vi "Desired Value Page.vi"(8 "error in (no error)":errorcluster, 11 "Node Ptr":T3 format="%.0x") -> (0 "error out":errorcluster)   [LabVIEW 2021, in "NI 272x Resistive Simulation Custom Device Configuration.lvlib"]
uses:
  NI 272x Resistive Simulation Custom Device Configuration.lvlib
  Program Files/National Instruments/LabVIEW 2021/vi.lib/NI VeriStand/Custom Device API/Custom Device Item Ref.ctl
  Program Files/National Instruments/LabVIEW 2021/instr.lib/ni272xReferenceVIs/ni272xReferenceVIs.llb/ni272x Callendar-Van Dusen RTD Parameters.ctl
  Controls/Channel Mode.ctl
  Globals/Names.vi
  Program Files/National Instruments/LabVIEW 2021/vi.lib/NI VeriStand/Custom Device API/Get Item Property (U16).vi
  Program Files/National Instruments/LabVIEW 2021/vi.lib/NI VeriStand/Custom Device API/Get Item Property (I32).vi
  Program Files/National Instruments/LabVIEW 2021/vi.lib/NI VeriStand/Custom Device API/Set Item Property (I32).vi
  Program Files/National Instruments/LabVIEW 2021/vi.lib/NI VeriStand/Custom Device API/Set Item Property (U16).vi
  Program Files/National Instruments/LabVIEW 2021/vi.lib/NI VeriStand/Custom Device API/Custom Device API.lvlib
  NI 272x Resistive Simulation Custom Device Shared.lvlib
panel:
  out "Units":string
  in  "Default Value":dbl
  in  "Mode":T1
  in  "Channel #":i32 min=0
  in  "Callendar-Van Dusen RTD parameters":T2={"A"=0.00139999995008111, "B"=0.00023700000019744039, "C"=9.899999753315569e-08, "R0"=1000.0}
  in  "Header":cluster{"Section Name":string}={"Section Name"="Desired Hardware Channel Value"}
  in  "Description":string
  in  "Name":string
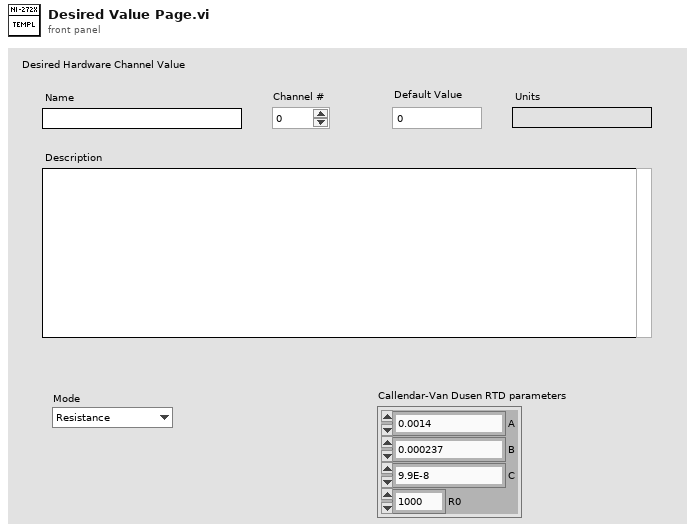
[diagram p1: front panel]
types:
  T1 = typedef "NI 272x Resistive Simulation Custom Device Shared.lvlib/Channel Mode.ctl" = enum16{"Resistance", "RTD Temperature"}
  T2 = typedef "ni272x Callendar-Van Dusen RTD Parameters.ctl" = cluster{"A":dbl, "B":dbl, "C":dbl, "R0":dbl}
  T3 = typedef "Custom Device API.lvlib/Custom Device Item Ref.ctl" = u64
  T4 = typedef "Custom Device API.lvlib/Custom Device Channel.ctl" = cluster{"Type":T5, "Units":string, "Default Value":dbl, "Faultable":bool, "Scalable":bool}
  T5 = typedef "Custom Device API.lvlib/Custom Device Channel Type.ctl" = enum16{"Input", "Output"}
  T6 = typedef "Custom Device API.lvlib/Custom Device Item Info.ctl" = cluster{"Name":string, "Is Channel":bool, "GUID":string, "Is Waveform":bool}
  T7 = typedef "Custom Device API.lvlib/Custom Device Commands.ctl" = enum16{"Default", "Item renamed", "Shutdown", "Dynamic button pressed"}
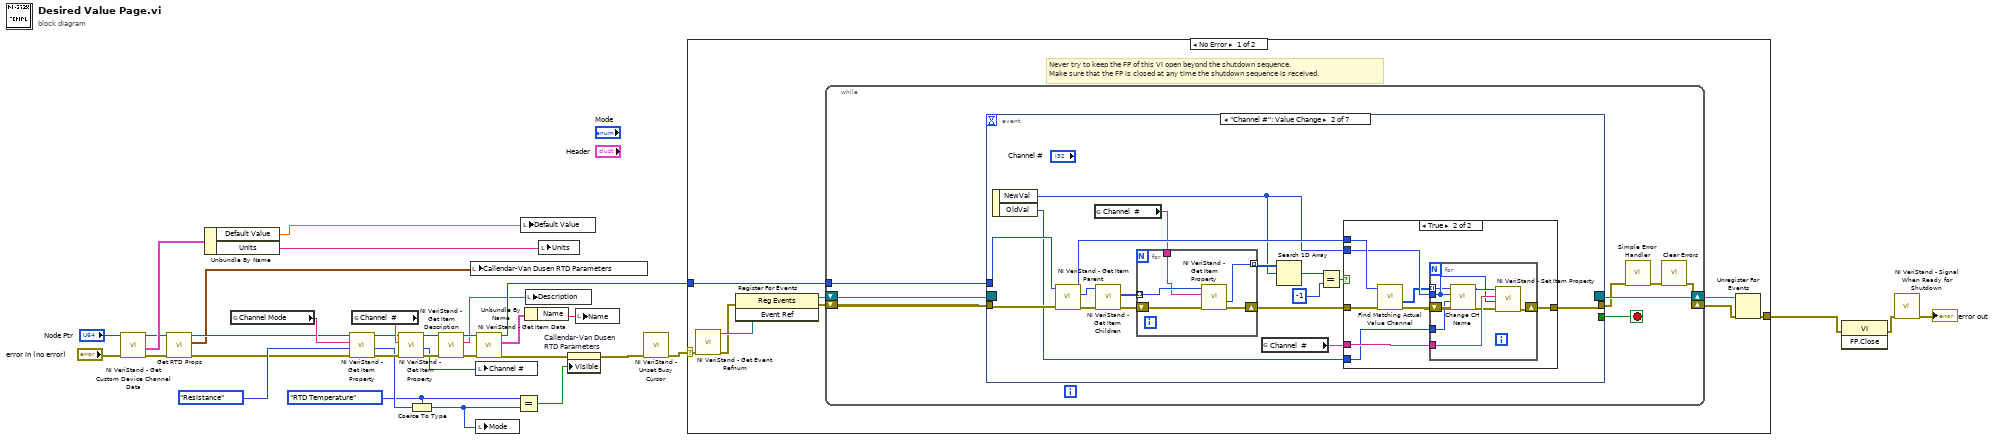
[diagram p0: block diagram]
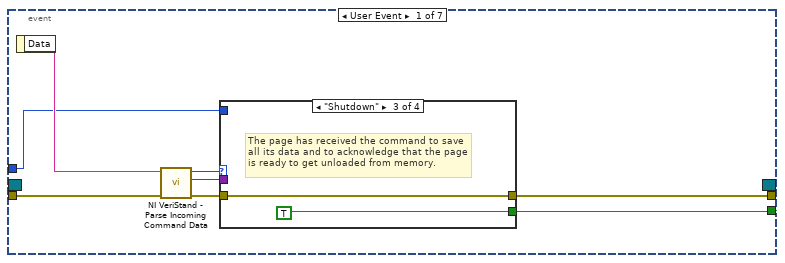
[diagram p2: hidden frame]
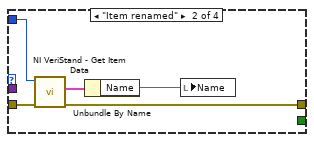
[diagram p4: hidden frame]
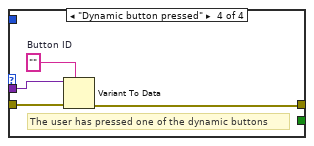
[diagram p5: hidden frame]
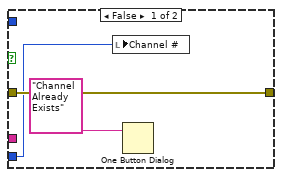
[diagram p6: hidden frame]
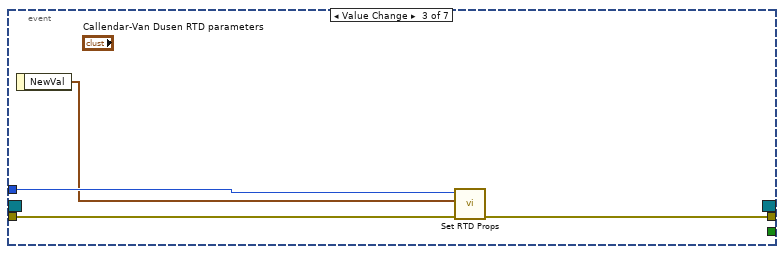
[diagram p7: hidden frame]
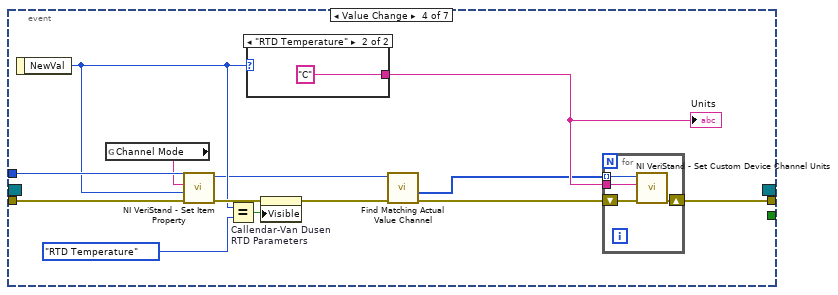
[diagram p8: hidden frame]
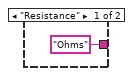
[diagram p9: hidden frame]
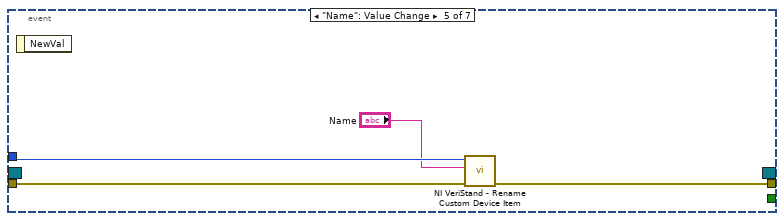
[diagram p10: hidden frame]
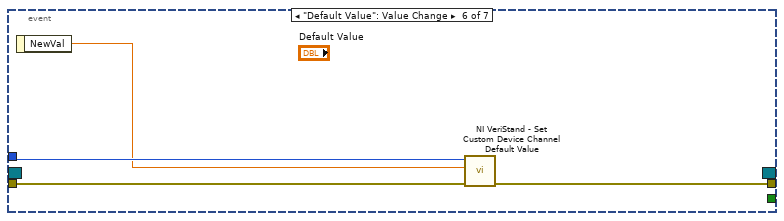
[diagram p11: hidden frame]
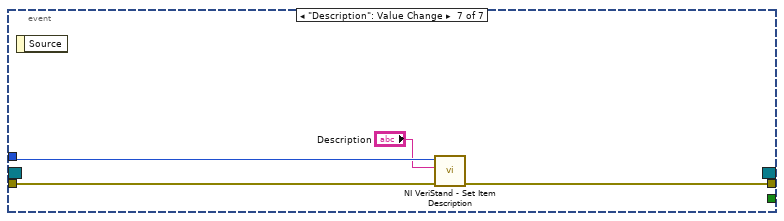
[diagram p12: hidden frame]
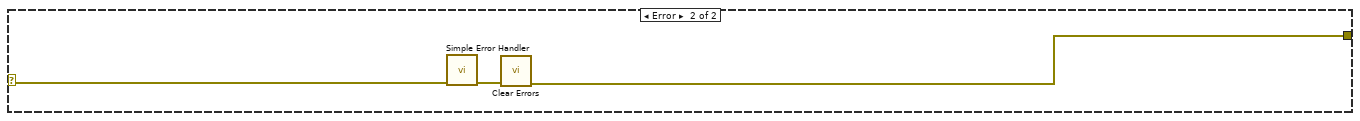
[diagram p13: hidden frame]
diagram:
  w13 = Channel_Mode."RTD Temperature" ("Mode")
  n1 = call "NI VeriStand - Get Custom Device Channel Data.vi"("error in (no error)"="error in (no error)", "Channel Ref in"="Node Ptr") -> ("error out"=w10:errorcluster, "Channel"=w8:T4, "Channel Ref out"=w3:T3)  [unwired: 4 in, 3 out]
  n2 = call "Get RTD Props.vi"("error in (no error)"=w10, "Item Ref in"=w3) -> ("error out"=w4:errorcluster, "temp param"=w1:T2, "Item Ref out"=w2:T3)  [unwired: 7 in]
  n3 = Unbundle By Name(w8) -> ("Default Value"=w5:dbl, "Units"=w7:string)
  n4 = global read "Names.vi" "Channel Mode"() -> (w16:string)
  n5 = call-poly "NI VeriStand - Get Item Property.vi"("error in (no error)"=w4, "Default Value"=Channel_Mode."Resistance" ("Mode"), "Property Name"=w16, "Item Ref in"=w2) -> ("error out"=w17:errorcluster, "Value"=w15:u16, "Item Ref out"=w18:T3)  [unwired: 4 in, 1 out]
  n6 = global read "Names.vi" "Channel  #"() -> (w20:string)
  n7 = call-poly "NI VeriStand - Get Item Property.vi"("error in (no error)"=w17, "Property Name"=w20, "Item Ref in"=w18) -> ("error out"=w21:errorcluster, "Value"=w19:i32, "Item Ref out"=w22:T3)  [unwired: 5 in, 1 out]
  n8 = Coerce To Type(0:w15, 1:w13) -> (2:w12:T1)
  n9 = call "NI VeriStand - Get Item Description.vi"("error in (no error)"=w21, "Item Ref in"=w22) -> ("error out"=w25:errorcluster, "Description"=w26:string, "Item Ref out"=w27:T3)  [unwired: 7 out]
  n10 = local write "Callendar-Van Dusen RTD parameters"(w1) -> ()
  n11 = local write "Channel #"(w19) -> ()
  n12 = local write "Mode"(w12) -> ()
  n13 = call "NI VeriStand - Get Item Data.vi"("error in (no error)"=w25, "Item Ref in"=w27) -> ("error out"=w14:errorcluster, "Item Info"=w24:T6, "Item Ref out"=w29:T3)  [unwired: 7 out]
  n14 = Equal?(x=w13, y=w12) -> (x = y?=w11:bool)
  n15 = local write "Default Value"(w5) -> ()
  n16 = Unbundle By Name(w24) -> ("Name"=w23:string)
  n17 = local write "Description"(w26) -> ()
  n18 = local write "Units"(w7) -> ()
  n19 = property on="Callendar-Van Dusen RTD Parameters" class="Clust (strict)"(error in=w14, "Visible"=w11) -> (error out=w31:errorcluster)  [unwired: 1 in, 1 out]
  n20 = local write "Name"(w23) -> ()
  n21 = call "NI VeriStand - Unset Busy Cursor.vi"("error in (no error)"=w31) -> ("error out"=w30:errorcluster)  [unwired: 10 out]
  n22 = case shown="No Error" w30 {
    selector: w30 -> [w36 w149]
    tunnel: [w41 w147] -> w34
    tunnel: w29 -> [w37 _]
    frame No Error {
      # "Never try to keep the FP of this VI open beyond the shutdown sequence.\nMake sure that the FP is closed at any time the shutdown sequence is received."
      n23 = call "NI VeriStand - Get Event Refnum.vi"("error in (no error)"=w36) -> ("error out"=w35:errorcluster, "Event Ref"=w40:refnum<user-event>)  [unwired: 9 out]
      n24 = register-events(error in=w35, w40) -> (reference out=w38:refnum<event-registration>, error out=w39:errorcluster)  [unwired: 1 in]
      n25 = while {
        tunnel: w37 -> [w47]
        shift-right: [w45] -> w42
        shift-left: w39 -> [w50]
        shift-right: [w51] -> w43
        shift-left: w38 -> [w49]
        stop <- w48 stop-if-true
        n26 = event shown="[1] \"Channel #\": Value Change" {
          selector: w49 -> [_ _ _ _ _ _ _]
          dyn-events: [_ _ _ _ _ _ _] -> w51
          timeout: _ -> [_ _ _ _ _ _ _]
          tunnel: w50 -> [w59 w78 w116 w128 w138 w142 w145]
          tunnel: [w55 _ _ _ _ _ _] -> w48
          tunnel: [w54 w74 w115 w122 w135 w140 w144] -> w44
          tunnel: w47 -> [w53 w77 w114 w127 w137 w141 w146]
          event User Event {
            n27 = event-data() -> ("Data"=w58:string)  [unwired: 1 out]
            n28 = call "NI VeriStand - Parse Incoming Command Data.vi"("error in (no error)"=w59, "Incoming data"=w58) -> ("error out"=w57:errorcluster, "Outgoing data"=w52:variant, "Action"=w56:T7)  [unwired: 7 out]
            n29 = case shown="\"Shutdown\"" w56 {
              tunnel: w57 -> [w60 w65 w66 w71]
              tunnel: [_ _ TRUE _] -> w55
              tunnel: [w60 w62 w66 w68] -> w54
              tunnel: w53 -> [_ w64 _ _]
              tunnel: w52 -> [_ _ _ w70]
              frame "Default", Default {
              }
              frame "Item renamed" {
                n30 = call "NI VeriStand - Get Item Data.vi"("error in (no error)"=w65, "Item Ref in"=w64) -> ("error out"=w62:errorcluster, "Item Info"=w63:T6)  [unwired: 8 out]
                n31 = Unbundle By Name(w63) -> ("Name"=w61:string)
                n32 = local write "Name"(w61) -> ()
              }
              frame "Shutdown" {
                # "The page has received the command to save all its data and to acknowledge that the page is ready to get unloaded from memory."
              }
              frame "Dynamic button pressed" {
                w69 = ""  # Button ID
                # "The user has pressed one of the dynamic buttons"
                n33 = Variant To Data(error in=w71, type=w69, Variant=w70) -> (error out=w68:errorcluster)  [unwired: 1 out]
              }
            }
          }
          event "Channel #": Value Change {
            n34 = event-data() -> ("NewVal"=w76:i32, "OldVal"=w75:i32)  [unwired: 1 out]
            n35 = call "NI VeriStand - Get Item Parent.vi"("error in (no error)"=w78, "Item Ref in"=w77) -> ("error out"=w79:errorcluster, "Parent Ref"=w80:T3, "Item Ref out"=w88:T3)  [unwired: 6 in, 1 out]
            n36 = global read "Names.vi" "Channel  #"() -> (w72:string)
            n37 = call "NI VeriStand - Get Item Children.vi"("error in (no error)"=w79, "Item Ref in"=w80) -> ("error out"=w82:errorcluster, "Child Refs"=w81:T3[])  [unwired: 6 in, 2 out]
            n38 = for {
              tunnel: w81 -> [w110] mode=indexing
              shift-right: [w111] -> w87
              shift-left: w82 -> [w112]
              tunnel: [w109] -> w83 mode=indexing
              tunnel: w72 -> [w108]
              n39 = call-poly "NI VeriStand - Get Item Property.vi"("error in (no error)"=w112, "Property Name"=w108, "Item Ref in"=w110) -> ("error out"=w111:errorcluster, "Value"=w109:i32)  [unwired: 5 in, 2 out]
            }
            n40 = global read "Names.vi" "Channel  #"() -> (w73:string)
            n41 = Search 1D Array(1D array=w83, element=w76) -> (index of element=w84:i32)  [unwired: 1 in]
            n42 = Equal?(x=w84, y=-1) -> (x = y?=w86:bool)
            n43 = case shown="True" w86 {
              tunnel: w87 -> [w91 w97]
              tunnel: w88 -> [_ w96]
              tunnel: w73 -> [_ w98]
              tunnel: w76 -> [_ w95]
              tunnel: [w91 w99] -> w74
              tunnel: w75 -> [w89 w92]
              frame False {
                n44 = local write "Channel #"(w89) -> ()
                n45 = One Button Dialog(message="Channel Already Exists") -> ()  [unwired: 1 in, 1 out]
              }
              frame True {
                n46 = call "Find Matching Actual Value Channel.vi"("error in (no error)"=w97, "Desired item ref in"=w96) -> ("error out"=w94:errorcluster, "Refs (desired first)"=w93:T3[])  [unwired: 4 in, 4 out]
                n47 = for {
                  tunnel: w98 -> [w106]
                  shift-right: [w107] -> w99
                  shift-left: w94 -> [w104]
                  tunnel: w95 -> [w102]
                  tunnel: w93 -> [w101] mode=indexing
                  tunnel: w92 -> [w100]
                  n48 = call "Change CH Name.vi"("error in (no error)"=w104, "Old #"=w100, "New #"=w102, "Node Ptr"=w101) -> ("error out"=w105:errorcluster, "Node Ptr out"=w103:T3)  [unwired: 6 in]
                  n49 = call-poly "NI VeriStand - Set Item Property.vi"("error in (no error)"=w105, "Value"=w102, "Property Name"=w106, "Item Ref in"=w103) -> ("error out"=w107:errorcluster)  [unwired: 5 in, 2 out]
                }
              }
            }
          }
          event Value Change {
            n50 = event-data() -> ("NewVal"=w113:T2)  [unwired: 1 out]
            n51 = call "Set RTD Props.vi"("error in (no error)"=w116, "temp param"=w113, "Item Ref in"=w114) -> ("error out"=w115:errorcluster)  [unwired: 7 in, 1 out]
          }
          event Value Change {
            n52 = event-data() -> ("NewVal"=w121:T1)  [unwired: 1 out]
            n53 = global read "Names.vi" "Channel Mode"() -> (w126:string)
            n54 = call-poly "NI VeriStand - Set Item Property.vi"("error in (no error)"=w128, "Value"=w121, "Property Name"=w126, "Item Ref in"=w127) -> ("error out"=w125:errorcluster, "Item Ref out"=w118:T3)  [unwired: 5 in, 1 out]
            n55 = Equal?(x=w121, y=Channel_Mode."RTD Temperature" ("NewVal")) -> (x = y?=w124:bool)
            n56 = case shown="\"RTD Temperature\"" w121 {
              tunnel: ["Ohms" ("Units") "C" ("Units")] -> w120
              frame "Resistance" {
              }
              frame "RTD Temperature" {
              }
            }
            "Units" <- w120
            n57 = property on="Callendar-Van Dusen RTD Parameters" class="Clust (strict)"(error in=w125, "Visible"=w124) -> (error out=w119:errorcluster)  [unwired: 1 in, 1 out]
            n58 = call "Find Matching Actual Value Channel.vi"("error in (no error)"=w119, "Desired item ref in"=w118) -> ("Refs (desired first)"=w117:T3[])  [unwired: 4 in, 5 out]
            n59 = for {
              tunnel: w120 -> [w131]
              shift-right: [w132] -> w122
              shift-left: w119 -> [w130]
              tunnel: w117 -> [w129] mode=indexing
              n60 = call "NI VeriStand - Set Custom Device Channel Units.vi"("error in (no error)"=w130, "Units"=w131, "Channel Ref in"=w129) -> ("error out"=w132:errorcluster)  [unwired: 7 in, 1 out]
            }
          }
          event "Name": Value Change {
            n61 = event-data() -> ()  [unwired: 2 out]
            n62 = call "NI VeriStand - Rename Custom Device Item.vi"("error in (no error)"=w138, "New Name"="Name", "Item Ref in"=w137) -> ("error out"=w135:errorcluster)  [unwired: 1 in, 7 out]
          }
          event "Default Value": Value Change {
            n63 = event-data() -> ("NewVal"=w139:dbl)  [unwired: 1 out]
            n64 = call "NI VeriStand - Set Custom Device Channel Default Value.vi"("error in (no error)"=w142, "Default Value"=w139, "Channel Ref in"=w141) -> ("error out"=w140:errorcluster)  [unwired: 7 in, 1 out]
          }
          event "Description": Value Change {
            n65 = event-data() -> ()  [unwired: 2 out]
            n66 = call "NI VeriStand - Set Item Description.vi"("error in (no error)"=w145, "Description"="Description", "Item Ref in"=w146) -> ("error out"=w144:errorcluster)  [unwired: 8 out]
          }
        }
        n67 = call <vilib>:"Simple Error Handler.vi"("error in (no error)"=w44) -> ("error out"=w46:errorcluster)  [unwired: 1 in, 7 out]
        n68 = call <vilib>:"Clear Errors.vi"("error in (no error)"=w46) -> ("error out"=w45:errorcluster)  [unwired: 1 in, 5 out]
      }
      n69 = Unregister For Events(event registration refnum=w43, error in=w42) -> (error out=w41:errorcluster)
    }
    frame Error {
      n70 = call <vilib>:"Simple Error Handler.vi"("error in (no error)"=w149) -> ("error out"=w148:errorcluster)  [unwired: 1 in, 7 out]
      n71 = call <vilib>:"Clear Errors.vi"("error in (no error)"=w148) -> ("error out"=w147:errorcluster)  [unwired: 1 in, 5 out]
    }
  }
  n72 = invoke class="VI" method="FP.Close"(error in=w34) -> (error out=w33:errorcluster)  [unwired: 2 in, 2 out]
  n73 = call "NI VeriStand - Signal When Ready for Shutdown.vi"("error in (no error)"=w33) -> ("error out"=→"error out":errorcluster)  [unwired: 10 out]
